vi "ziGetEventCntSample.vi"(8 "Error In":errorcluster, 10 "Cnt Sample In":T1, 11 "Handle In":T2 {"Handle" format="0x%08x"; "Conn" format="0x%08x"}) -> (0 "Error Out":errorcluster, 2 "Cnt Sample Out":T1, 3 "Handle Out":T2 {"Handle" format="0x%08x"; "Conn" format="0x%08x"})   [LabVIEW 2015, in "Zurich Instruments LabOne.lvlib"]
uses:
  Zurich Instruments LabOne.lvlib
  Zurich Instruments/LabOne/API/LabVIEW/Zurich Instruments LabOne/Private/ziLV64.framework
  ziTypeHandle.ctl
  ziTypeCounterSample.ctl
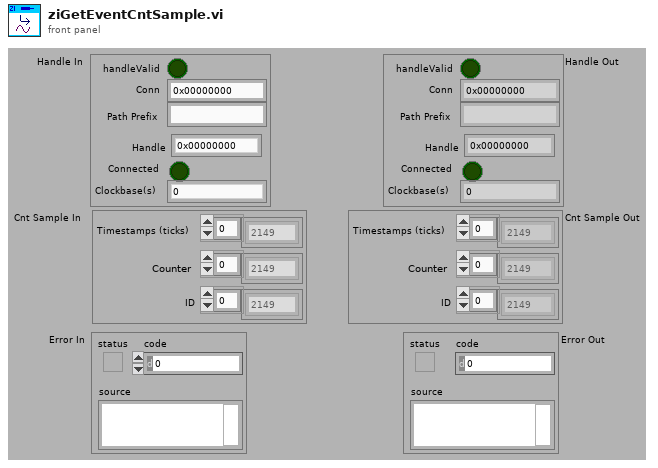
[diagram p1: front panel]
types:
  T1 = typedef "Zurich Instruments LabOne.lvlib/ziTypeCounterSample.ctl" = cluster{"Timestamps (ticks)":u64[], "Counter":i32[], "ID":u16[]}
  T2 = typedef "Zurich Instruments LabOne.lvlib/ziTypeHandle.ctl" = cluster{"handleValid":bool, "Conn":u64, "Path Prefix":string, "Handle":u64, "Connected":bool, "Clockbase(s)":dbl}
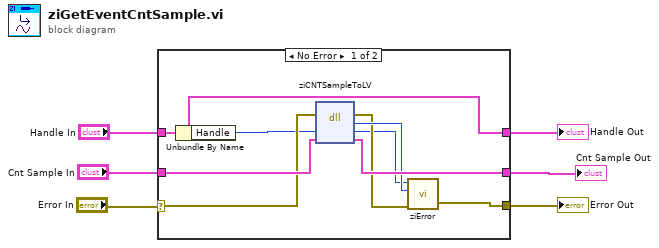
[diagram p0: block diagram]
diagram:
  n1 = case shown="No Error" "Error In" {
    selector: "Error In" -> [w12 w16]
    tunnel: "Handle In" -> [w8 w18]
    tunnel: [w8 w18] -> w5
    tunnel: [w15 w17] -> w4
    tunnel: "Cnt Sample In" -> [w14 w17]
    tunnel: [w13 w16] -> w2
    frame No Error {
      n2 = Unbundle By Name(w8) -> ("Handle"=w11:u64)
      n3 = dll-call lib="Users/arkady/Desktop/ado/github/resonant_ultrasound_arxiv/maglab ultrasound -- arkady --arxiv/Zurich Instruments/LabOne/API/LabVIEW/Zurich Instruments LabOne/Private/ziLV*.*" fn="ziCNTSampleToLV"(error in=w12, "ziEventBuffer"=w11, "ImpSample"=w14) -> (error out=w9:errorcluster, "return type"=w10:u32, "ziEventBuffer"=w7:u64, "ImpSample"=w15:T1)  [unwired: 2 in, 1 out]
      n4 = call "ziError.vi"("Conn"=w7, "ziErrorCode"=w10, "Error In"=w9) -> ("Error Out"=w13:errorcluster)  [unwired: 2 in, 1 out]
    }
    frame Error {
    }
  }
  "Handle Out" <- w5
  "Error Out" <- w2
  "Cnt Sample Out" <- w4
